vi "DEMO Factory.vi"() -> ()   [LabVIEW 2019]
uses:
  Generic Plugin/Plugin Type.ctl
  Generic Plugin/Generic Plugin.lvclass
panel:
  in  "stop":bool
  out "Plugin Color":u32(colorbox)
  out "Plugin says:":string
  in  "Plugin type":T1
  # "change the enum to various values to see what each class says.\nsee block diagram for comments"
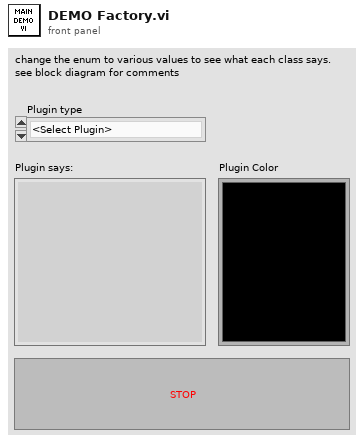
[diagram p1: front panel]
types:
  T1 = typedef "Generic Plugin.lvclass/Plugin Type.ctl" = enum16{"<Select Plugin>", "Orange", "Blue", "Red"}
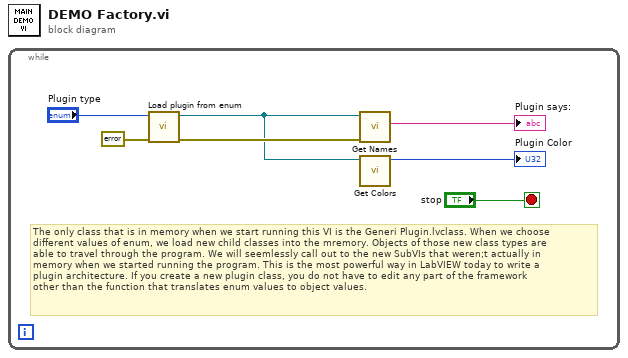
[diagram p0: block diagram]
diagram:
  n1 = while {
    stop <- "stop" stop-if-true
    # "The only class that is in memory when we start running this VI is the Generi Plugin.lvclass. When we choose\ndifferent values of enum, we load new child classes into the mremory. Objects of those new class types are\nable to travel through the program. We will seemlessly call out to the new SubVIs that weren;t actually in\nmemory when we started running the program. This is the most powerful way in LabVIEW today to write a \nplugin architecture. If you create a new plugin class, you do not have to edit any part of the framework\nother than the function that translates enum values to object values."
    n2 = call "Load plugin from enum.vi"("error in (no error)"=errorcluster {"status"=FALSE, "code"=0, "source"=""}, "Plugin type"="Plugin type") -> ("error out"=w4:errorcluster, "Generic Plugin out"=w2:refnum<class "Generic Plugin.lvclass">)  [unwired: 4 in]
    n3 = call-dynamic "Get Names.vi"("error in (no error)"=w4, "Generic Plugin in"=w2) -> ("Name"=→"Plugin says:":string)  [unwired: 7 in, 2 out]
    n4 = call-dynamic "Get Colors.vi"("Generic Plugin in"=w2) -> ("Color Box"=→"Plugin Color":u32)  [unwired: 10 in]
  }
